vi "Node Informations.vi"(8 "error in (no error)":errorcluster, 11 "String":string) -> (0 "error out":errorcluster, 1 "YAML Internal Type":T1, 2 "Value":string, 3 "Key":string, 4 "Level":u32)   [LabVIEW 2015, in "YAML Parser.lvclass"]
uses:
  YAML Parser.lvclass
  YAML Internal Type.ctl
panel:
  out "has Key?":bool
  out "key empty?":bool
  out "value empty?":bool
  out "length":i32
  out "Spaces Before Key":string
  out "First Char":string
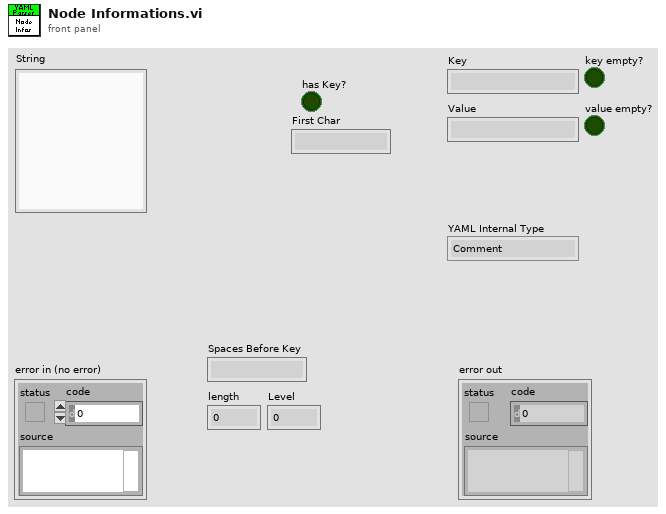
[diagram p1: front panel]
types:
  T1 = typedef "YAML Parser.lvclass/YAML Internal Type.ctl" = enum16{"Comment", "Null", "Value", "Multilines Value", "Object", "Array", "Reference", "Array Element", "Empty Line", "Key"}
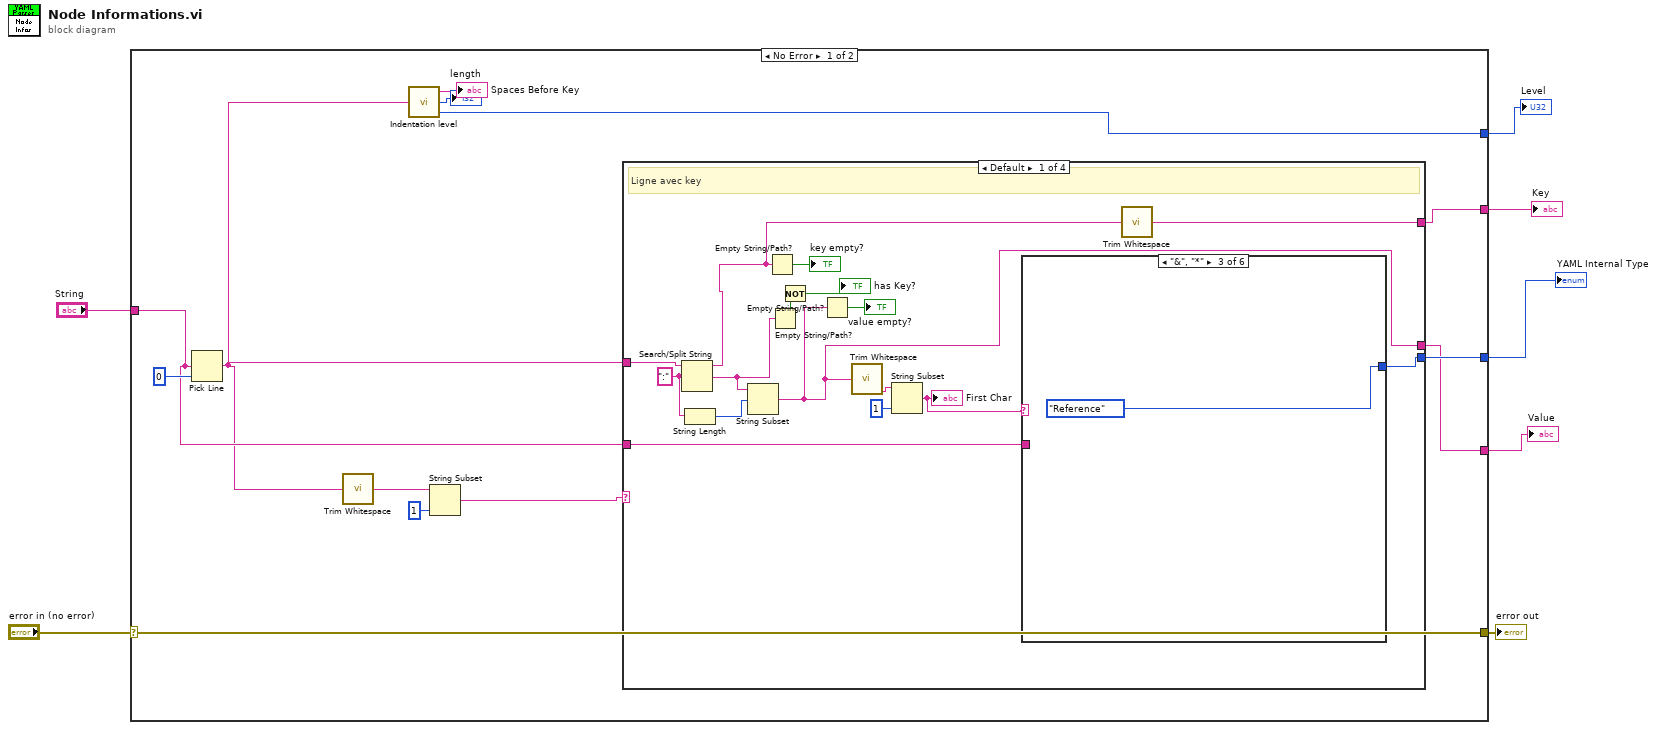
[diagram p0: block diagram]
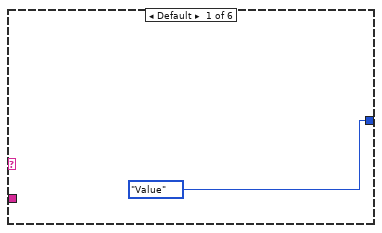
[diagram p2: hidden frame]
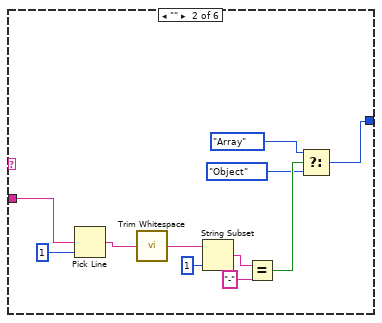
[diagram p3: hidden frame]
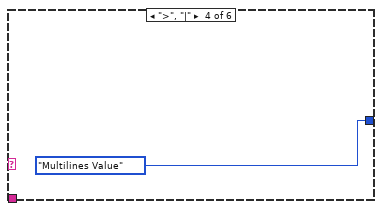
[diagram p4: hidden frame]
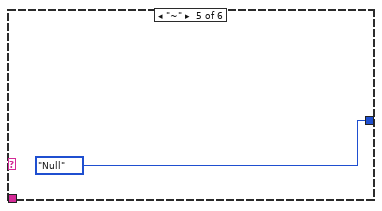
[diagram p5: hidden frame]
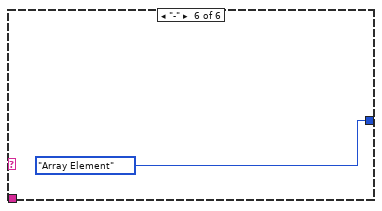
[diagram p6: hidden frame]
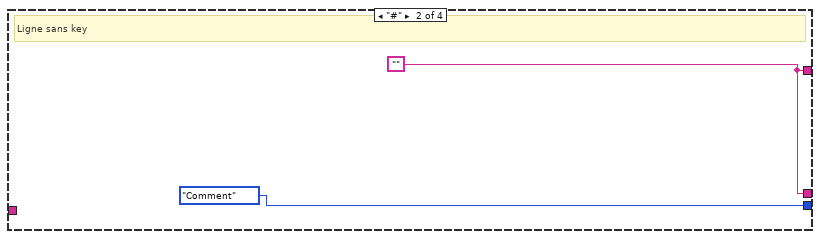
[diagram p7: hidden frame]
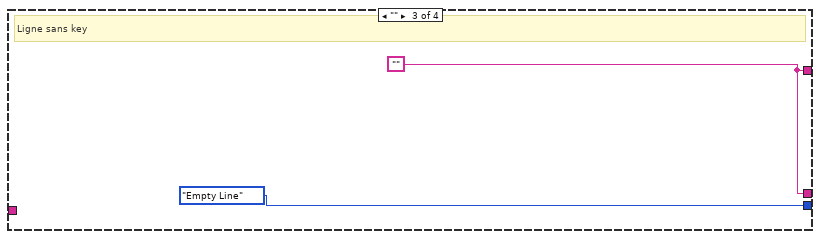
[diagram p8: hidden frame]
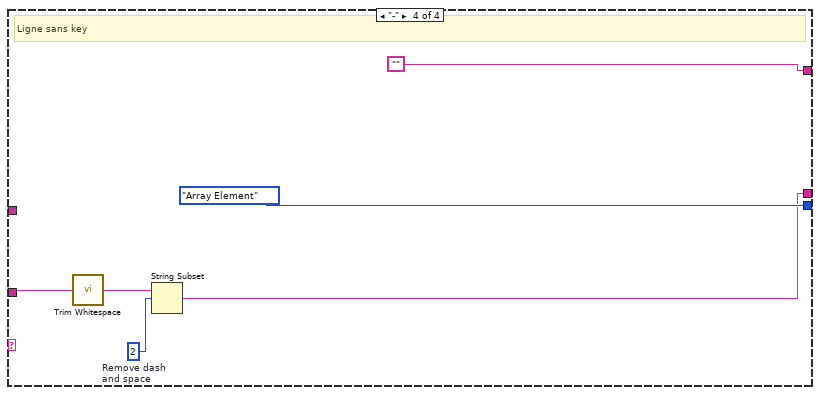
[diagram p9: hidden frame]
diagram:
  n1 = case shown="No Error" "error in (no error)" {
    selector: "error in (no error)" -> [w20 w63]
    tunnel: [w20 w63] -> w6
    tunnel: "String" -> [w13 _]
    tunnel: [w19 _] -> w4
    tunnel: [w14 _] -> w3
    tunnel: [w10 _] -> w2
    tunnel: [w9 _] -> w1
    frame No Error {
      n2 = Pick Line(multi-line string=w13, line index=0) -> (output string=w8:string)  [unwired: 1 in]
      n3 = call <vilib>:"Trim Whitespace.vi"("string"=w8) -> ("trimmed string"=w11:string)  [unwired: 1 in]
      n4 = call "Indentation level.vi"("String"=w8) -> ("Spaces Before Key"=→"Spaces Before Key":string, "length"=→"length":i32, "Level"=w14:u32)
      n5 = String Subset(string=w11, length (rest)=1 ("length (rest)")) -> (substring=w12:string)  [unwired: 1 in]
      n6 = case shown="Default" w12 {
        tunnel: [w36 YAML_Internal_Type."Comment" ("YAML Internal Type") YAML_Internal_Type."Empty Line" ("YAML Internal Type") YAML_Internal_Type."Array Element" ("YAML Internal Type")] -> w19
        tunnel: w13 -> [w35 _ _ w60]
        tunnel: [w34 w54 w56 ""] -> w9
        tunnel: [w21 w54 w56 w58] -> w10
        tunnel: w8 -> [w22 _ _ _]
        frame Default {
          w28 = ":" ("search string/char (-)")
          # "Ligne avec key"
          n7 = Search/Split String(string=w22, search string/char (-)=w28) -> (substring before match=w23:string, match + rest of string=w31:string)  [unwired: 1 in, 1 out]
          n8 = String Length(string=w28) -> (length=w27:i32)
          n9 = String Subset(string=w31, offset (0)=w27) -> (substring=w21:string)  [unwired: 1 in]
          n10 = Empty String/Path?(string/path=w23) -> (empty?=→"key empty?":bool)
          n11 = Empty String/Path?(string/path=w31) -> (empty?=w32:bool)
          n12 = Not(x=w32) -> (.not. x?=→"has Key?":bool)
          n13 = Empty String/Path?(string/path=w21) -> (empty?=→"value empty?":bool)
          n14 = call <vilib>:"Trim Whitespace.vi"("string"=w21) -> ("trimmed string"=w25:string)  [unwired: 1 in]
          n15 = String Subset(string=w25, length (rest)=1 ("length (rest)")) -> (substring=w24:string)  [unwired: 1 in]
          "First Char" <- w24
          n16 = case shown="\"&\", \"*\"" w24 {
            tunnel: [YAML_Internal_Type."Value" ("YAML Internal Type") w38 YAML_Internal_Type."Reference" ("YAML Internal Type") YAML_Internal_Type."Multilines Value" ("YAML Internal Type") YAML_Internal_Type."Null" ("YAML Internal Type") YAML_Internal_Type."Array Element" ("YAML Internal Type")] -> w36
            tunnel: w35 -> [_ w47 _ _ _ _]
            frame Default {
            }
            frame "" {
              n17 = Pick Line(multi-line string=w47, line index=1) -> (output string=w46:string)  [unwired: 1 in]
              n18 = call <vilib>:"Trim Whitespace.vi"("string"=w46) -> ("trimmed string"=w45:string)  [unwired: 1 in]
              n19 = String Subset(string=w45, length (rest)=1 ("length (rest)")) -> (substring=w43:string)  [unwired: 1 in]
              n20 = Equal?(x=w43, y="-") -> (x = y?=w41:bool)
              n21 = Select(t=YAML_Internal_Type."Array" ("YAML Internal Type"), s=w41, f=YAML_Internal_Type."Object" ("YAML Internal Type")) -> (s? t:f=w38:T1)
            }
            frame "&", "*" {
            }
            frame ">", "|" {
            }
            frame "~" {
            }
            frame "-" {
            }
          }
          n22 = call <vilib>:"Trim Whitespace.vi"("string"=w23) -> ("trimmed string"=w34:string)  [unwired: 1 in]
        }
        frame "#" {
          w54 = ""
          # "Ligne sans key"
        }
        frame "" {
          w56 = ""
          # "Ligne sans key"
        }
        frame "-" {
          w57 = 2  # Remove dash and space
          # "Ligne sans key"
          n23 = call <vilib>:"Trim Whitespace.vi"("string"=w60) -> ("trimmed string"=w59:string)  [unwired: 1 in]
          n24 = String Subset(string=w59, offset (0)=w57) -> (substring=w58:string)  [unwired: 1 in]
        }
      }
    }
    frame Error {
    }
  }
  "error out" <- w6
  "YAML Internal Type" <- w4
  "Level" <- w3
  "Key" <- w1
  "Value" <- w2
